vi "Ej_5_Variables_locales.vi"() -> ()   [LabVIEW 2021]
panel:
  in  "Boolean 2":bool
  out "Waveform Chart 2":dbl(graph)
  out "Waveform Chart":dbl(graph)
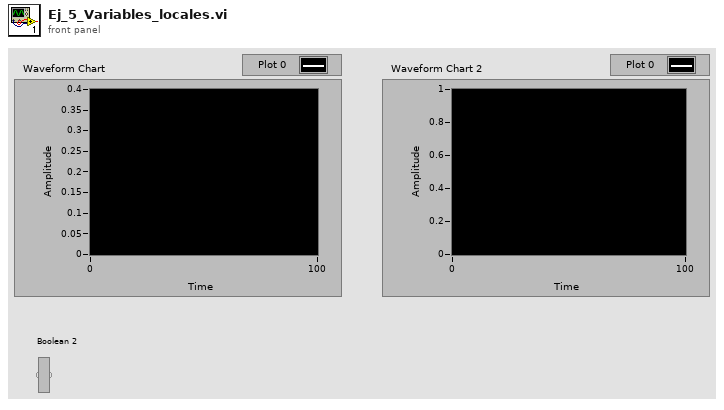
[diagram p1: front panel]
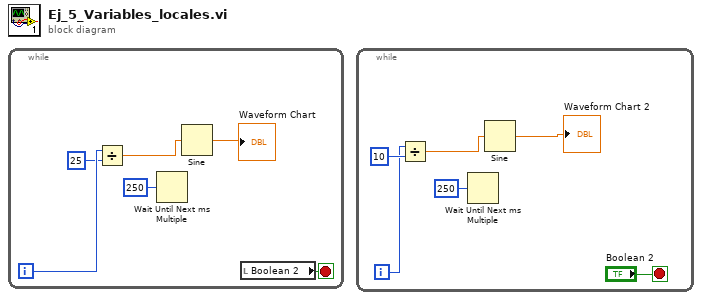
[diagram p0: block diagram]
diagram:
  n1 = while {
    i -> [w5]
    stop <- w1 stop-if-true
    n2 = Divide(x=w5, y=25) -> (x/y=w6:dbl)
    n3 = Wait Until Next ms Multiple(millisecond multiple=u32 250) -> ()  [unwired: 1 out]
    n4 = Sine(x=w6) -> (sin(x)=→"Waveform Chart":dbl)
    n5 = local read "Boolean 2"() -> (w1:bool)
  }
  n6 = while {
    i -> [w10]
    stop <- "Boolean 2" stop-if-true
    n7 = Divide(x=w10, y=10) -> (x/y=w12:dbl)
    n8 = Wait Until Next ms Multiple(millisecond multiple=u32 250) -> ()  [unwired: 1 out]
    n9 = Sine(x=w12) -> (sin(x)=→"Waveform Chart 2":dbl)
  }
